vi "Constructor from Column.vi"(8 "error in (no error)":errorcluster, 10 "Column":refnum<class "Composed Column.lvclass">, 11 "Composed Field in":refnum<class "Composed Field.lvclass">) -> (0 "error out":errorcluster, 3 "Composed Field out":refnum<class "Composed Field.lvclass">)   [LabVIEW 2020, in "Composed Fields.lvlib" / "Composed Field.lvclass"]
uses:
  Composed Field.lvclass
  C:/Users/User/Desktop/Raman Program/Database OOP/source/Database OOP/Column Libraries/Column/Composed Column.lvclass
  Column/Composed Column.lvclass
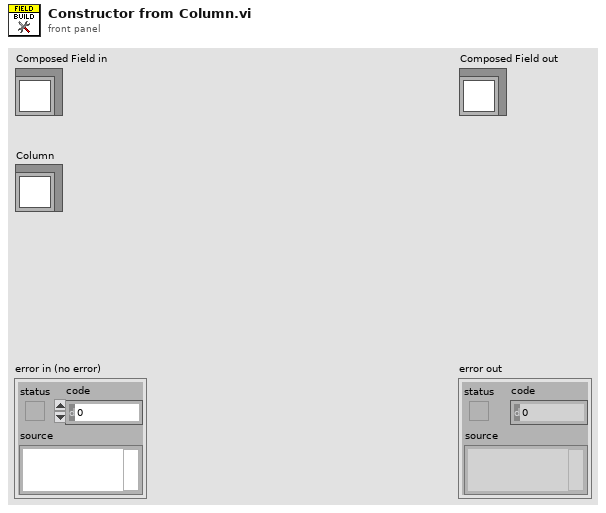
[diagram p1: front panel]
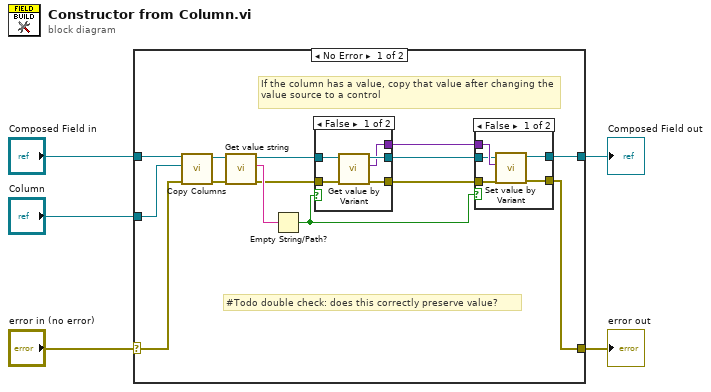
[diagram p0: block diagram]
diagram:
  n1 = case shown="No Error" "error in (no error)" {
    selector: "error in (no error)" -> [w17 w35]
    tunnel: [w8 w35] -> w4
    tunnel: [w9 w34] -> w2
    tunnel: "Composed Field in" -> [w19 w34]
    tunnel: "Column" -> [w18 _]
    frame No Error {
      # "#Todo double check: does this correctly preserve value?"
      # "If the column has a value, copy that value after changing the value source to a control"
      n2 = call "Copy Columns.vi"("error in (no error)"=w17, "Copy Column"=w18, "New Column Type"=w19) -> ("error out"=w15:errorcluster, "New Column Out"=w16:refnum<class "Composed Field.lvclass">)  [unwired: 7 in]
      n3 = call-dynamic "Get value string.vi"("error in (no error)"=w15, "Column in"=w16) -> ("error out"=w12:errorcluster, "Value"=w14:string, "Column out"=w13:refnum<class "Composed Field.lvclass">)  [unwired: 7 in]
      n4 = Empty String/Path?(string/path=w14) -> (empty?=w11:bool)
      n5 = case shown="False" w11 {
        tunnel: w13 -> [w31 w33]
        tunnel: w12 -> [w30 w32]
        tunnel: [w29 w33] -> w7
        tunnel: [w28 w32] -> w6
        tunnel: [w27 _] -> w10
        frame False {
          n6 = call-dynamic "Get value by Variant.vi"("error in (no error)"=w30, "Column in"=w31) -> ("error out"=w28:errorcluster, "Variant"=w27:variant, "Column out"=w29:refnum<class "Composed Field.lvclass">)  [unwired: 7 in]
        }
        frame True {
        }
      }
      n7 = case shown="False" w11 {
        tunnel: w7 -> [w23 w26]
        tunnel: w6 -> [w22 w25]
        tunnel: w10 -> [w24 _]
        tunnel: [w21 w26] -> w9
        tunnel: [w20 w25] -> w8
        frame False {
          n8 = call-dynamic "Set value by Variant.vi"("error in (no error)"=w22, "Variant"=w24, "Column in"=w23) -> ("error out"=w20:errorcluster, "Column out"=w21:refnum<class "Composed Field.lvclass">)  [unwired: 7 in]
        }
        frame True {
        }
      }
    }
    frame Error {
    }
  }
  "error out" <- w4
  "Composed Field out" <- w2
